vi "Midpoint Circle.vi"() -> ()   [LabVIEW 2017]
panel:
  out "XY Graph":cluster{i32[], i32[]}(graph)
  out "transposed array":cluster{"X":i32, "Y":i32}[][](array[cluster])
  out "Decreasing Order (3-7-1-5)":cluster{"X":i32, "Y":i32}[][](array[cluster])
  out "Increasing Order (2-6-4-8)":cluster{"X":i32, "Y":i32}[][](array[cluster])
  out "Pixels":cluster{"X":i32, "Y":i32}[][](array[cluster])
  in  "(Xc, Yc)":cluster{"Xc":i32, "Yc":i32}
  in  "Radius":i32
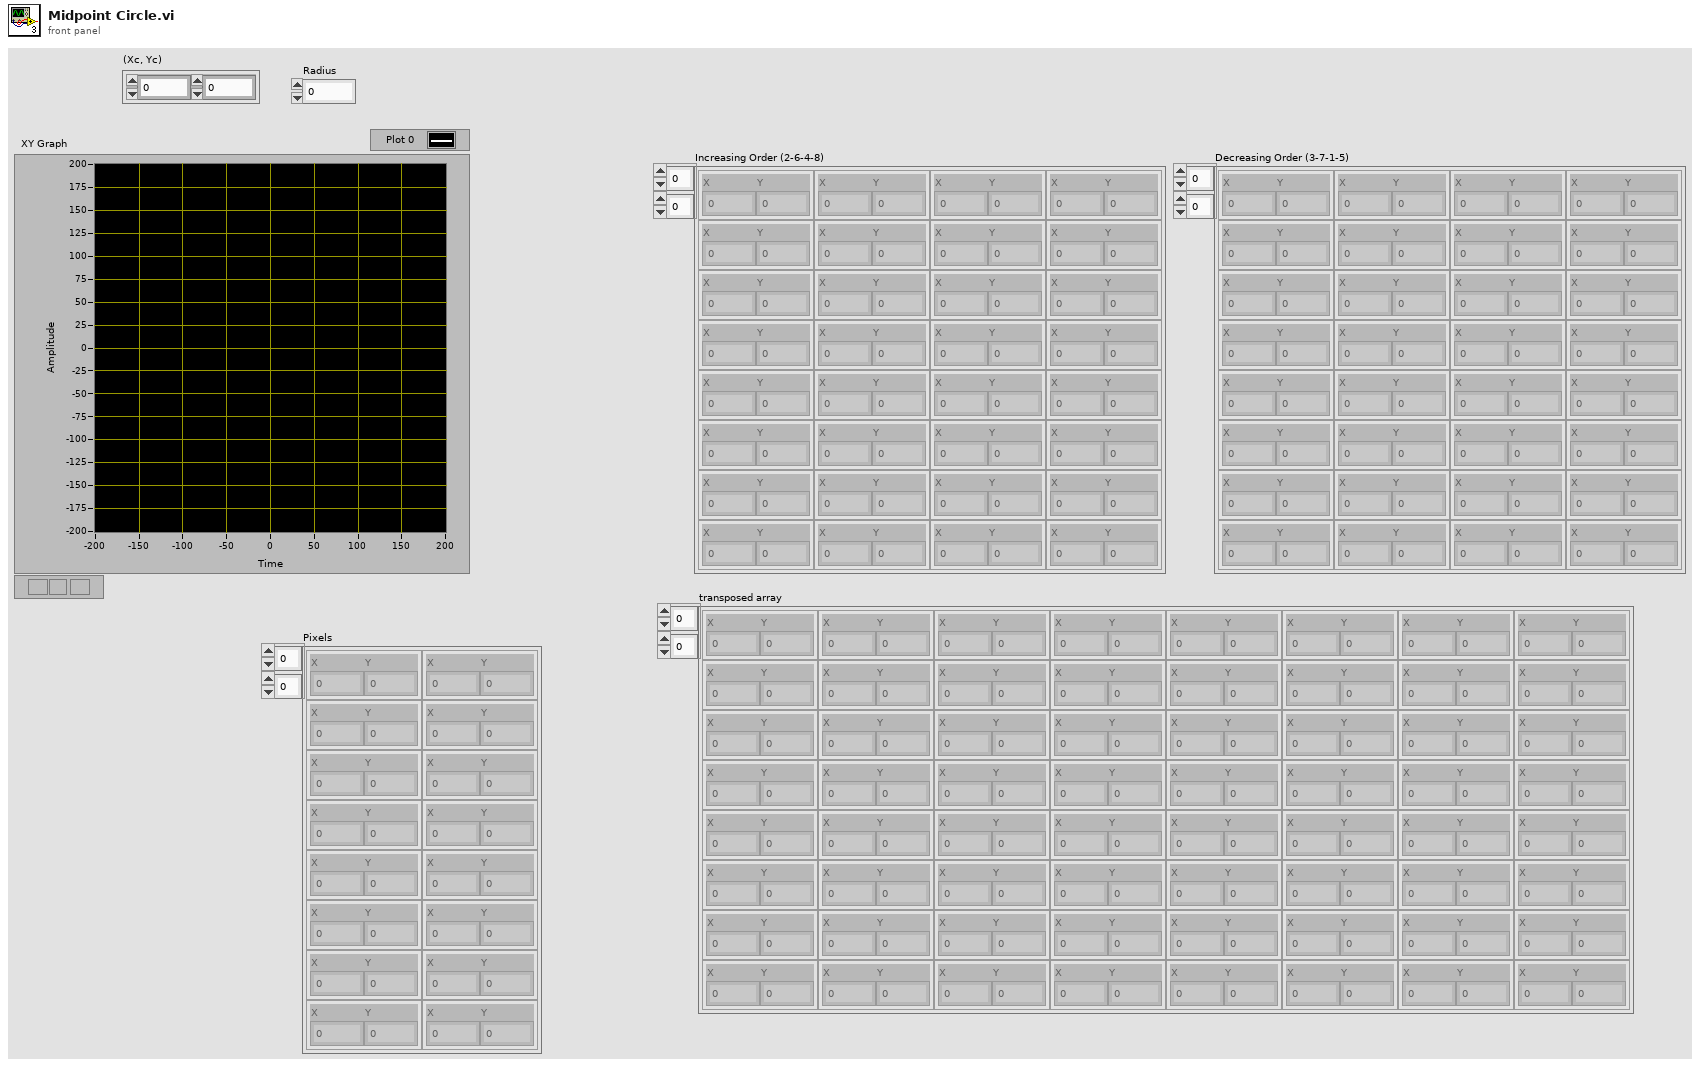
[diagram p1: front panel]
types:
  T1 = cluster{"k":i32, "Pk":i32, "Xk+1":i32, "Yk+1":i32}[]
  T2 = cluster{"k":i32, "Pk":i32, "Xk+1":i32, "Yk+1":i32}
  T3 = enum16{"Full", "Half", "Quarter", "Eighth", "Sixteenth"}
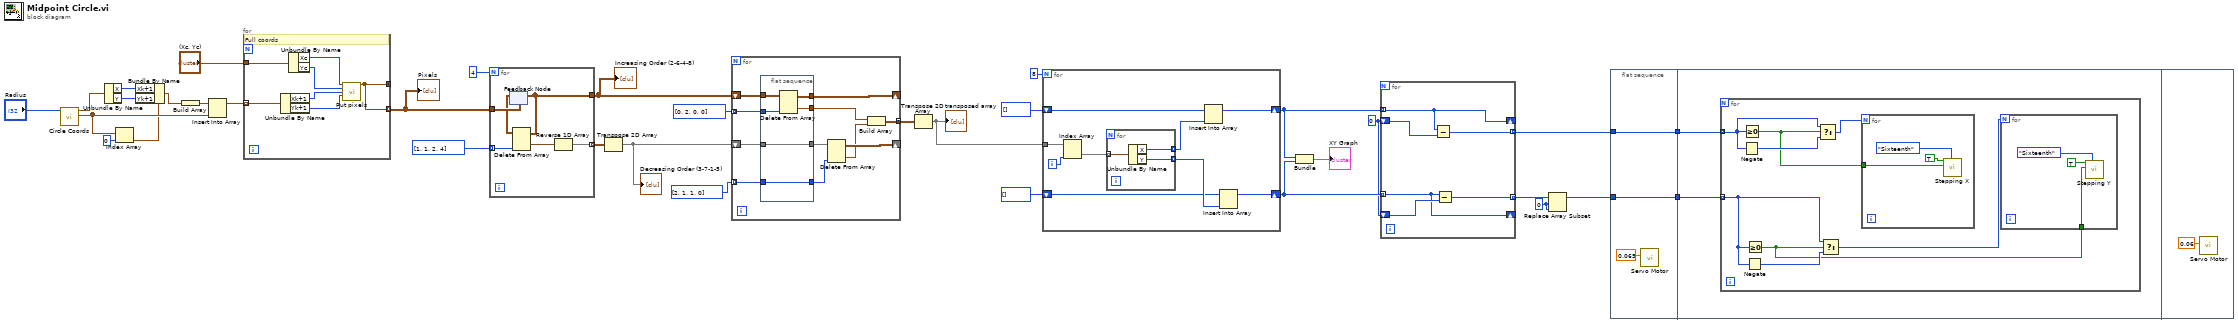
[diagram p0: block diagram]
diagram:
  w1 = 0 ("index")
  w9 = 0 ("X")
  n1 = call "Circle Coords.vi"("Radius"="Radius") -> ("Coordinates"=w31:T1, "Init coord"=w27:cluster{"X":i32, "Y":i32})  [unwired: 8 in, 1 out]
  n2 = Unbundle By Name(w27) -> ("X"=w26:i32, "Y"=w25:i32)
  n3 = Index Array(array=w31, index=0) -> (element=w30:T2)
  n4 = Bundle By Name(cluster=w30, "Xk+1"=w26, "Yk+1"=w25) -> (w29:T2)
  n5 = Build Array(w29) -> (w28:T1)
  n6 = Insert Into Array(array=w28, new element=w31) -> (w32:T1)  [unwired: 1 in]
  n7 = for {
    tunnel: w32 -> [w41] mode=indexing
    tunnel: "(Xc, Yc)" -> [w40]
    tunnel: [w35] -> _ mode=concatenating
    tunnel: [w35] -> w23 mode=indexing
    # "Full coords"
    n8 = Unbundle By Name(w41) -> ("Xk+1"=w36:i32, "Yk+1"=w37:i32)
    n9 = Unbundle By Name(w40) -> ("Xc"=w39:i32, "Yc"=w38:i32)
    n10 = call "Put pixels.vi"("Xc"=w39, "Yc"=w38, "X"=w36, "Y"=w37) -> ("Pixels"=w35:cluster{"X":i32, "Y":i32}[])  [unwired: 10 in, 1 out]
  }
  "Pixels" <- w23
  n11 = for {
    N: 4 -> [_]
    tunnel: w23 -> [w47]
    tunnel: [w45] -> w19
    tunnel: i32[] [1, 1, 2, 4] -> [w44] mode=indexing
    tunnel: [w43] -> w20 mode=indexing
    n12 = feedback #1(w47) -> (w46:cluster{"X":i32, "Y":i32}[][])
    n13 = Delete From Array(array=w46, index (col)=w44) -> (deleted portion=w42:cluster{"X":i32, "Y":i32}[], array with subset deleted=w45:cluster{"X":i32, "Y":i32}[][])  [unwired: 2 in]
    n14 = feedback-in #1(w45) -> ()
    n15 = Reverse 1D Array(array=w42) -> (reversed array=w43:cluster{"X":i32, "Y":i32}[])
  }
  "Increasing Order (2-6-4-8)" <- w19
  n16 = Transpose 2D Array(2D array=w20) -> (transposed array=w18:cluster{"X":i32, "Y":i32}[][])
  "Decreasing Order (3-7-1-5)" <- w18
  n17 = for {
    shift-right: [w58] -> _
    shift-left: w18 -> [w53]
    shift-right: [w56] -> _
    shift-left: w19 -> [w57]
    tunnel: i32[] [2, 1, 1, 0] -> [w51] mode=indexing
    tunnel: i32[] [0, 2, 0, 0] -> [w55] mode=indexing
    tunnel: [w48] -> w15 mode=concatenating
    n18 = flat-sequence {
      tunnel: w57 -> [w64]
      tunnel: [w63] -> w50
      tunnel: [w62] -> w56
      tunnel: w55 -> [w61]
      tunnel: w53 -> [w60]
      tunnel: [w60] -> w54
      tunnel: [w59] -> w52
      tunnel: w51 -> [w59]
      frame #0 {
        n19 = Delete From Array(array=w64, index (col)=w61) -> (deleted portion=w63:cluster{"X":i32, "Y":i32}[], array with subset deleted=w62:cluster{"X":i32, "Y":i32}[][])  [unwired: 2 in]
      }
    }
    n20 = Delete From Array(array=w54, index (col)=w52) -> (deleted portion=w49:cluster{"X":i32, "Y":i32}[], array with subset deleted=w58:cluster{"X":i32, "Y":i32}[][])  [unwired: 2 in]
    n21 = Build Array(w50, w49) -> (w48:cluster{"X":i32, "Y":i32}[][])
  }
  n22 = Transpose 2D Array(2D array=w15) -> (transposed array=w14:cluster{"X":i32, "Y":i32}[][])
  "transposed array" <- w14
  n23 = for {
    N: 8 -> [_]
    tunnel: w14 -> [w73]
    shift-right: [w69] -> w11
    shift-left: i32[] [] -> [w68]
    shift-right: [w66] -> w10
    shift-left: i32[] [] -> [w65]
    i -> [w72]
    n24 = Index Array(array=w73, index (col)=w72) -> (element=w71:cluster{"X":i32, "Y":i32}[])  [unwired: 1 in]
    n25 = for {
      tunnel: [w75] -> w67 mode=indexing
      tunnel: [w74] -> w70 mode=indexing
      tunnel: w71 -> [w76] mode=indexing
      n26 = Unbundle By Name(w76) -> ("X"=w74:i32, "Y"=w75:i32)
    }
    n27 = Insert Into Array(array=w68, new element=w70) -> (w69:i32[])  [unwired: 1 in]
    n28 = Insert Into Array(array=w65, new element=w67) -> (w66:i32[])  [unwired: 1 in]
  }
  n29 = Bundle(w11, w10) -> (→"XY Graph":cluster{i32[], i32[]})  [unwired: 1 in]
  n30 = for {
    tunnel: w11 -> [w82] mode=indexing
    shift-right: [w82] -> _
    shift-left: w9 -> [w81]
    tunnel: [w80] -> w4 mode=indexing
    tunnel: w10 -> [w78] mode=indexing
    shift-right: [w78] -> _
    shift-left: w9 -> [w79]
    tunnel: [w77] -> w2 mode=indexing
    n31 = Subtract(x=w82, y=w81) -> (x-y=w80:i32)
    n32 = Subtract(x=w78, y=w79) -> (x-y=w77:i32)
  }
  n33 = Replace Array Subset(array=w2, new element=w1, index=w1) -> (w3:i32[])
  n34 = flat-sequence {
    tunnel: w3 -> [w84]
    tunnel: w4 -> [w85]
    tunnel: [w85] -> w8
    tunnel: [w84] -> w7
    tunnel: w8 -> [w87]
    tunnel: w7 -> [w86]
    frame #0 {
      n35 = call "Servo Motor.vi"("Duty Cycle"=0.065) -> ()  [unwired: 9 in, 2 out]
    }
    frame #1 {
      n36 = for {
        tunnel: w87 -> [w93] mode=indexing
        tunnel: w86 -> [w90] mode=indexing
        n37 = Negate(x=w93) -> (-x=w94:i32)
        n38 = Greater Or Equal To 0?(x=w93) -> (x >= 0?=w92:bool)
        n39 = Negate(x=w90) -> (-x=w91:i32)
        n40 = Greater Or Equal To 0?(x=w90) -> (x >= 0?=w88:bool)
        n41 = Select(t=w93, s=w92, f=w94) -> (s? t:f=w95:i32)
        n42 = Select(t=w90, s=w88, f=w91) -> (s? t:f=w89:i32)
        n43 = for {
          N: w95 -> [_]
          tunnel: w92 -> [w99]
          n44 = call "Stepping X.vi"("Microstep size"=T3."Sixteenth", "Direction"=w99, "Enable"=TRUE) -> ()  [unwired: 8 in, 1 out]
        }
        n45 = for {
          N: w89 -> [_]
          tunnel: w88 -> [w96]
          n46 = call "Stepping Y.vi"("Microstep size"=T3."Sixteenth", "Direction"=w96, "Enable"=TRUE) -> ()  [unwired: 8 in, 1 out]
        }
      }
    }
    frame #2 {
      n47 = call "Servo Motor.vi"("Duty Cycle"=0.06) -> ()  [unwired: 9 in, 2 out]
    }
  }
